vi "Ejemplo.vi"(2 "PathImagen":path, 3 "Original":T1) -> (0 "AreaHerida":dbl, 1 "Mask":T1)   [LabVIEW 2021]
uses:
  <vilib>/vision/Image Controls.llb/IMAQ Image.ctl
  <vilib>/Utility/file.llb/Read Delimited Spreadsheet (string).vi
  <vilib>/Utility/file.llb/Write Delimited Spreadsheet (string).vi
  <vilib>/vision/NI_Vision_Development_Module.lvlib
panel:
  out "Image Out":T1
  out "Image Dst Out":T1
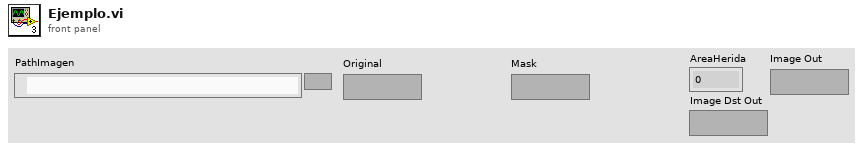
[diagram p1: front panel]
types:
  T1 = typedef "IMAQ Image.ctl" = refnum<image>
  T2 = typedef "Particle Parameters" = i32
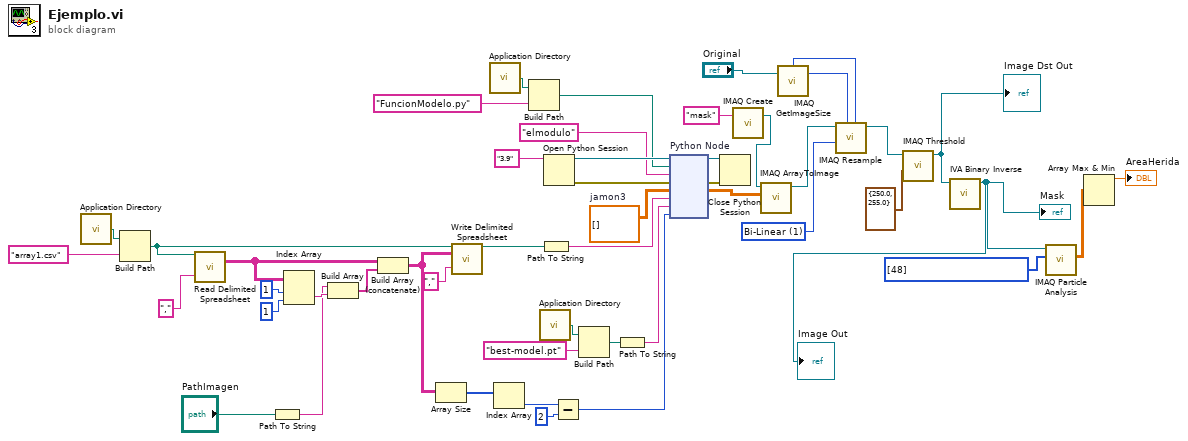
[diagram p0: block diagram]
diagram:
  w6 = T2[] [48] items=["Center of Mass X", "Center of Mass Y", "First Pixel X", "First Pixel Y", "Bounding Rect Left", "Bounding Rect Top", "Bounding Rect Right", "Bounding Rect Bottom", "Max Feret Diameter Start X", "Max Feret Diameter Start Y", "Max Feret Diameter End X", "Max Feret Diameter End Y", "Max Horiz. Segment Length Left", "Max Horiz. Segment Length Right", "Max Horiz. Segment Length Row", "-", "Bounding Rect Width", "Bounding Rect Height", "Bounding Rect Diagonal", "Perimeter", "Convex Hull Perimeter", "Holes' Perimeter", "Max Feret Diameter", "Equivalent Ellipse Major Axis", "Equivalent Ellipse Minor Axis", "Equivalent Ellipse Minor Axis (Feret)", "Equivalent Rect Long Side", "Equivalent Rect Short Side", "Equivalent Rect Diagonal", "Equivalent Rect Short Side (Feret)", "Average Horiz. Segment Length", "Average Vert. Segment Length", "Hydraulic Radius", "Waddel Disk Diameter", "-", "Area", "Holes' Area", "Particle & Holes' Area", "Convex Hull Area", "Image Area", "-", "Number of Holes", "Number of Horiz. Segments", "Number of Vert. Segments", "-", "Orientation", "Max Feret Diameter Orientation", "-", "% Area/Image Area", "% Area/(Particle & Holes' Area)", "Ratio of Equivalent Ellipse Axes", "Ratio of Equivalent Rect Sides", "-", "Elongation Factor", "Compactness Factor", "Heywood Circularity Factor", "Type Factor", "-", "Sum X", "Sum Y", "Sum XX", "Sum XY", "Sum YY", "Sum XXX", "Sum XXY", "Sum XYY", "Sum YYY", "-", "Moment of Inertia XX", "Moment of Inertia XY", "Moment of Inertia YY", "Moment of Inertia XXX", "Moment of Inertia XXY", "Moment of Inertia XYY", "Moment of Inertia YYY", "Norm. Moment of Inertia XX", "Norm. Moment of Inertia XY", "Norm. Moment of Inertia YY", "Norm. Moment of Inertia XXX", "Norm. Moment of Inertia XXY", "Norm. Moment of Inertia XYY", "Norm. Moment of Inertia YYY", "Hu Moment 1", "Hu Moment 2", "Hu Moment 3", "Hu Moment 4", "Hu Moment 5", "Hu Moment 6", "Hu Moment 7"] ("Pixel Measurements")
  w39 = u32 1 items=["Zero Order", "Bi-Linear", "Quadratic", "Cubic Spline"] ("Interpolation Type")
  w43 = dbl[][] []  # jamon3
  n1 = call <vilib>:"Application Directory.vi"() -> ("Application Directory"=w13:path)
  n2 = Build Path(base path=w13, name or relative path="array1.csv") -> (appended path=w12:path)
  n3 = call-poly <vilib>:"Read Delimited Spreadsheet.vi"("file path (dialog if empty)"=w12, "delimiter (\\t)"="," ("delimiter (\\t)")) -> ("all rows"=w28:string[][])  [unwired: 8 in, 5 out]
  n4 = Path To String(path="PathImagen") -> (string=w25:string)
  n5 = Index Array "Index Array"(array=w28, index (row)=1 ("disabled index (row)"), index (col)=1 ("disabled index (col)")) -> (element=w26:string)
  n6 = Build Array "Build Array"(w25, w26) -> (w27:string[])
  n7 = Build Array (concatenate)(w28, w27) -> (w19:string[][])
  n8 = Array Size(array=w19) -> (size(s)=w29:i32[])
  n9 = call-poly <vilib>:"Write Delimited Spreadsheet.vi"("file path (dialog if empty)"=w12, "2D data"=w19, "delimiter (\\t)"="," ("delimiter (\\t)")) -> ("new file path (Not A Path if cancelled)"=w18:path)  [unwired: 11 in, 1 out]
  n10 = call <vilib>:"Application Directory.vi"() -> ("Application Directory"=w10:path)
  n11 = Index Array(array=w29) -> (element=w30:i32)  [unwired: 1 in]
  n12 = Build Path(base path=w10, name or relative path="FuncionModelo.py") -> (appended path=w9:path)
  n13 = call <vilib>:"Application Directory.vi"() -> ("Application Directory"=w17:path)
  n14 = Path To String(path=w18) -> (string=w33:string)
  n15 = Open Python Session(python version="3.9" ("Python version")) -> (session out=w48:refnum<k35>, error out=w46:errorcluster)  [unwired: 2 in]
  n16 = Subtract(x=w30, y=2) -> (x-y=w21:i32)
  n17 = Build Path(base path=w17, name or relative path="best-model.pt") -> (appended path=w15:path)
  n18 = Path To String(path=w15) -> (string=w32:string)
  n19 = node "Python Node"(w48, w9, "elmodulo" ("function name"), w46, w43, w33, w32, w21) -> (w47:refnum<k35>, w45:errorcluster, w42:dbl[][])  [unwired: 3 in, 2 out]
  n20 = Close Python Session(session in=w47, error in=w45) -> ()  [unwired: 1 out]
  n21 = call "IMAQ Create"("Image Name"="mask") -> ("New Image"=w41:T1)  [unwired: 4 in, 1 out]
  n22 = call "IMAQ ArrayToImage"("Image Pixels (U8)"=w42, "Image"=w41) -> ("Image Out"=w34:T1)  [unwired: 8 in, 1 out]
  n23 = call "IMAQ GetImageSize"("Image"="Original") -> ("Y Resolution"=w36:i32, "X Resolution"=w35:i32)  [unwired: 3 in, 1 out]
  n24 = call "IMAQ Resample"("X Resolution"=w35, "Y Resolution"=w36, "Interpolation Type"=w39, "Image Src"=w34) -> ("Image Dst Out"=w37:T1)  [unwired: 6 in, 1 out]
  n25 = call "IMAQ Threshold"("Range"=cluster{"Lower value":sgl, "Upper value":sgl} {"Lower value"=250.0, "Upper value"=255.0}, "Image Src"=w37) -> ("Image Dst Out"=w7:T1)  [unwired: 8 in, 1 out]
  "Image Dst Out" <- w7
  n26 = call <vilib>:"IVA Binary Inverse.vi"("Image In"=w7) -> ("Image Out"=w1:T1)  [unwired: 1 in, 9 out]
  "Mask" <- w1
  "Image Out" <- w1
  n27 = call "IMAQ Particle Analysis"("Pixel Measurements"=w6, "Image"=w1) -> ("Particle Measurements (Pixels)"=w5:dbl[][])  [unwired: 4 in, 5 out]
  n28 = Array Max & Min(array=w5) -> (max value=→"AreaHerida":dbl)  [unwired: 3 out]
